vi "EEI EXP7.vi"() -> ()   [LabVIEW 2020]
panel:
  out "MIN 1D array":i32
  out "MAX 1D array":i32
  out "Array":i32[](array[numeric])
  out "EVEN no.s":i32[](array[numeric])
  out "current time":timestamp
  in  "no of even no.s":i32
  out "2D Array using for loop":dbl[][](array[numeric])
  in  "No. of columns":i32
  in  "No. of rows":i32
  out "1D Array using for loop":dbl[](array[numeric])
  in  "No. of random numbers":i32
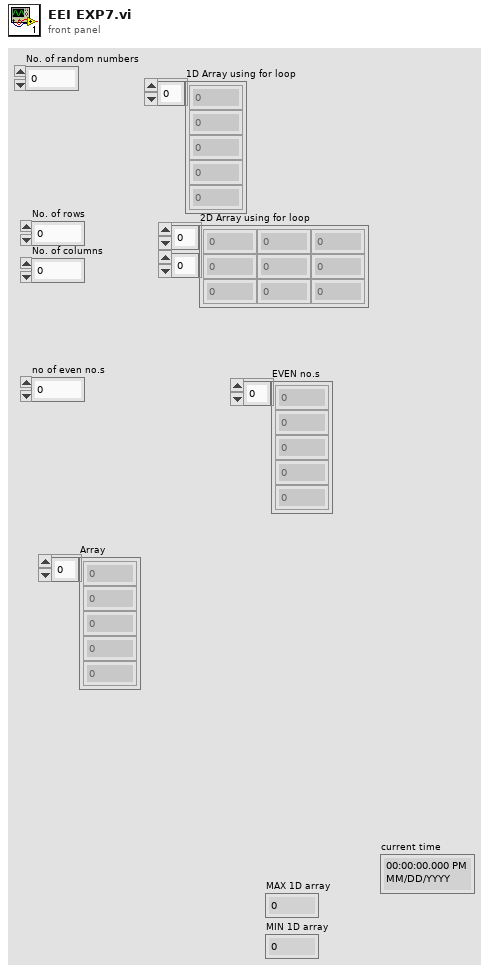
[diagram p1: front panel]
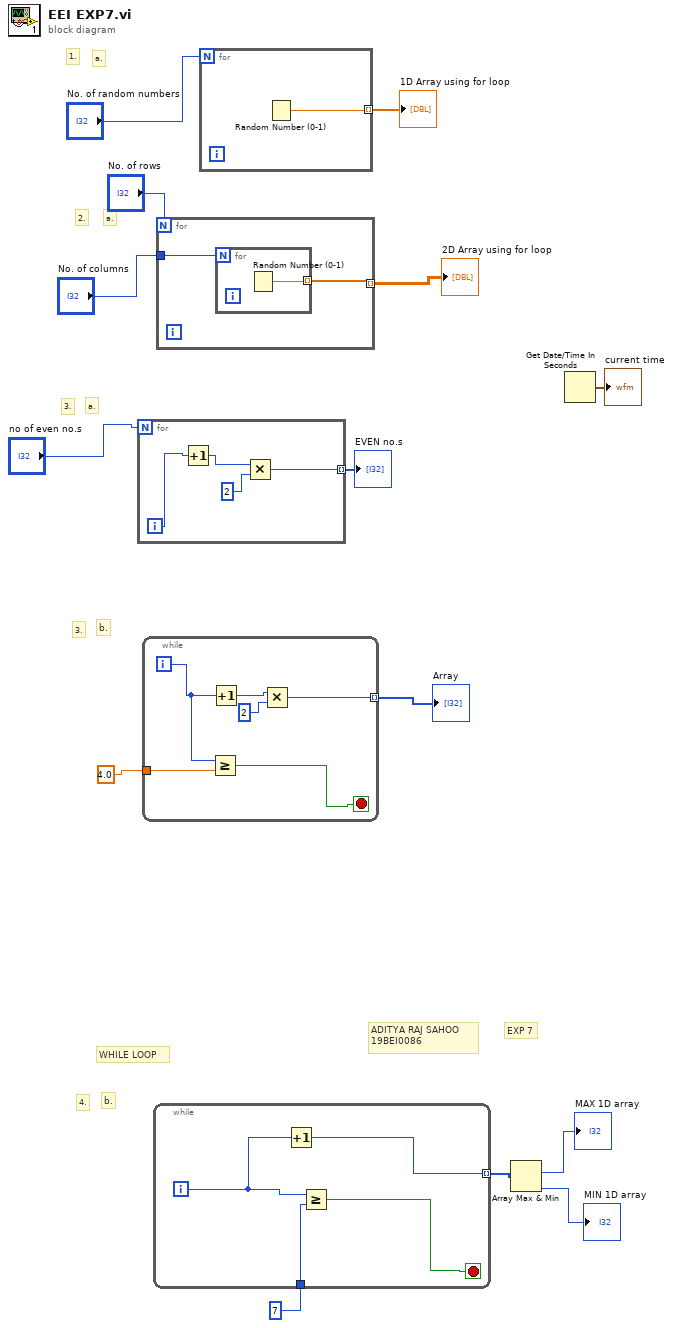
[diagram p0: block diagram]
diagram:
  # "WHILE LOOP"
  # "b."
  # "4."
  # "b."
  # "3."
  # "a."
  # "3."
  # "a."
  # "2."
  # "1."
  # "a."
  # "EXP 7"
  # "ADITYA RAJ SAHOO\n19BEI0086"
  n1 = for {
    N: "no of even no.s" -> [_]
    tunnel: [w15] -> w7 mode=indexing
    i -> [w18]
    n2 = Increment(x=w18) -> (x+1=w17:i32)
    n3 = Multiply(x=w17, y=2) -> (x*y=w15:i32)
  }
  "EVEN no.s" <- w7
  n4 = while {
    tunnel: 4.0 ("y") -> [w22]
    tunnel: [w19] -> w5 mode=indexing
    i -> [w21]
    stop <- w23 stop-if-true
    n5 = Greater Or Equal?(x=w21, y=w22) -> (x >= y?=w23:bool)
    n6 = Increment(x=w21) -> (x+1=w24:i32)
    n7 = Multiply(x=w24, y=2) -> (x*y=w19:i32)
  }
  "Array" <- w5
  n8 = while {
    tunnel: [w26] -> w4 mode=indexing
    tunnel: 7 ("x") -> [w25]
    i -> [w27]
    stop <- w28 stop-if-true
    n9 = Increment(x=w27) -> (x+1=w26:i32)
    n10 = Greater Or Equal?(x=w27, y=w25) -> (x >= y?=w28:bool)
  }
  n11 = for {
    N: "No. of rows" -> [_]
    tunnel: "No. of columns" -> [w30]
    tunnel: [w29] -> w10 mode=indexing
    n12 = for {
      N: w30 -> [_]
      tunnel: [w31] -> w29 mode=indexing
      n13 = Random Number (0-1)() -> (number: 0 to 1=w31:dbl)
    }
  }
  "2D Array using for loop" <- w10
  n14 = for {
    N: "No. of random numbers" -> [_]
    tunnel: [w32] -> w13 mode=indexing
    n15 = Random Number (0-1)() -> (number: 0 to 1=w32:dbl)
  }
  "1D Array using for loop" <- w13
  n16 = Array Max & Min(array=w4) -> (max index (indices)=→"MAX 1D array":i32, min index (indices)=→"MIN 1D array":i32)  [unwired: 2 out]
  n17 = Get Date/Time In Seconds() -> (seconds since 1Jan1904=→"current time":timestamp)
